vi "SPARK Get Status 0.vi"(8 "error in (no error)":errorcluster, 11 "MotorControlDevRef":T2) -> (0 "error out":errorcluster, 2 "Status 0":T1, 3 "MotorControlDevRef":T2)   [LabVIEW 2023]
uses:
  Typedef/Spark MAX Variant Data.ctl
  Typedef/SPARK Model.ctl
  Typedef/SPARK CAN Arb ID.ctl
  Typedef/SPARK Status 0 Frame.ctl
  <vilib>/Rock Robotics/SystemInterfaces/DIO/FPGA_DIOPWMChannel.ctl
  <vilib>/Rock Robotics/WPI/PWM/WPI_PWMDeadband.ctl
  <vilib>/Rock Robotics/WPI/MotorControl/WPI_MotorControlType.ctl
  <vilib>/Rock Robotics/SystemInterfaces/DIO/FPGA_DIOChannel.ctl
  <vilib>/Rock Robotics/WPI/MotorControl/WPI_MotorControlDeviceRef.ctl
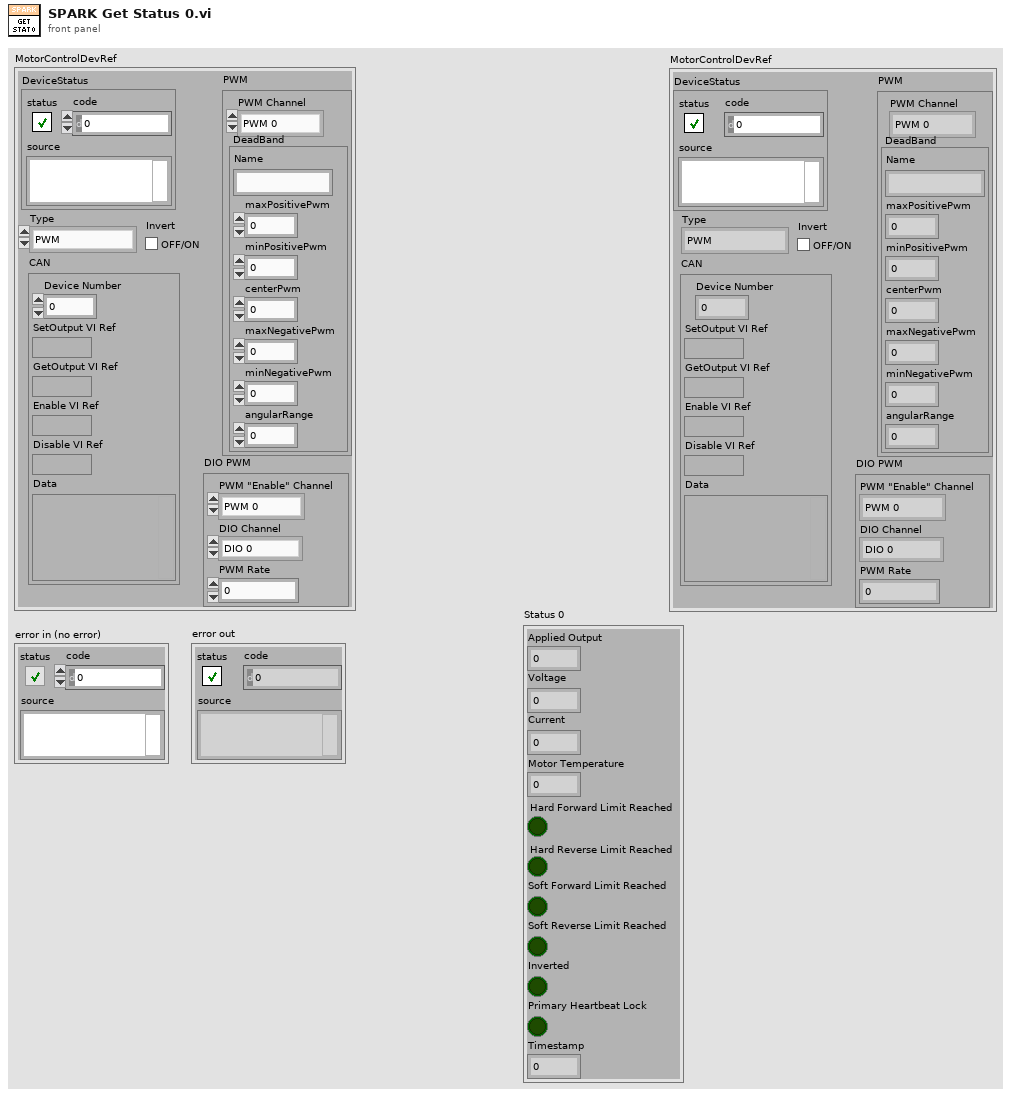
[diagram p1: front panel]
types:
  T1 = typedef "SPARK Status 0 Frame.ctl" = cluster{"Applied Output":dbl, "Voltage":dbl, "Current":dbl, "Motor Temperature":u8, "Hard Forward Limit Reached":bool, "Hard Reverse Limit Reached":bool, "Soft Forward Limit Reached":bool, "Soft Reverse Limit Reached":bool, "Inverted":bool, "Primary Heartbeat Lock":bool, "Timestamp":u32}
  T2 = typedef "WPI_MotorControlDeviceRef.ctl" = cluster{"DeviceStatus":errorcluster, "Type":T3, "PWM":cluster{"PWM Channel":T4, "DeadBand":T5}, "CAN":cluster{"Device Number":u8, "SetOutput VI Ref":variant, "GetOutput VI Ref":variant, "Enable VI Ref":variant, "Disable VI Ref":variant, "Data":variant}, "Invert":bool, "DIO PWM":cluster{"PWM \"Enable\" Channel":T4, "DIOChannel":T6, "PWM Rate":dbl}}
  T3 = typedef "WPI_MotorControlType.ctl" = enum16{"PWM", "CAN", "DIO PWM"}
  T4 = typedef "FPGA_DIOPWMChannel.ctl" = enum8{"PWM 0", "PWM 1", "PWM 2", "PWM 3", "PWM 4", "PWM 5", "PWM 6", "PWM 7", "PWM 8", "PWM 9", "PWM MXP 0", "PWM MXP 1", "PWM MXP 2", "PWM MXP 3", "PWM MXP 4", "PWM MXP 5", "PWM MXP 6", "PWM MXP 7", "PWM MXP 8", "PWM MXP 9", "Invalid"}
  T5 = typedef "WPI_PWMDeadband.ctl" = cluster{"Name":string, "maxPositivePwm":i32, "minPositivePwm":i32, "centerPwm":i32, "maxNegativePwm":i32, "minNegativePwm":i32, "angularRange":u16}
  T6 = typedef "FPGA_DIOChannel.ctl" = enum8{"DIO 0", "DIO 1", "DIO 2", "DIO 3", "DIO 4", "DIO 5", "DIO 6", "DIO 7", "DIO 8", "DIO 9", "DIO MXP 0", "DIO MXP 1", "DIO MXP 2", "DIO MXP 3", "DIO MXP 4", "DIO MXP 5", "DIO MXP 6", "DIO MXP 7", "DIO MXP 8", "DIO MXP 9", "DIO MXP 10", "DIO MXP 11", "DIO MXP 12", "DIO MXP 13", "DIO MXP 14", "DIO MXP 15", "SPI Port CS1", "SPI Port CS2", "SPI Port CS3", "SPI Port MISO", "SPI Port MOSI", "Invalid"}
  T7 = typedef "SPARK CAN Arb ID.ctl" = u32
  T8 = typedef "Spark MAX Variant Data.ctl" = cluster{"Ext ID":u32, "CAN Timeout":u32, "Inverted No WPILib":bool, "Has Configured Limit Sw":bool, "Has Configured Alt Encoder":bool, "SPARK Model":T9, "CAN Max Retries":u32, "CAN Timeout (ms)":u32, "Status 0 Period (ms)":u32, "Status 1 Period (ms)":u32, "Status 2 Period (ms)":u32, "Status 3 Period (ms)":u32, "Status 4 Period (ms)":u32, "Status 5 Period (ms)":u32, "Status 6 Period (ms)":u32, "Status 7 Period (ms)":u32, "Status Frame Timeout (ms)":u32}
  T9 = typedef "SPARK Model.ctl" = enum16{"SPARK MAX", "SPARK Flex", "Unknown"}
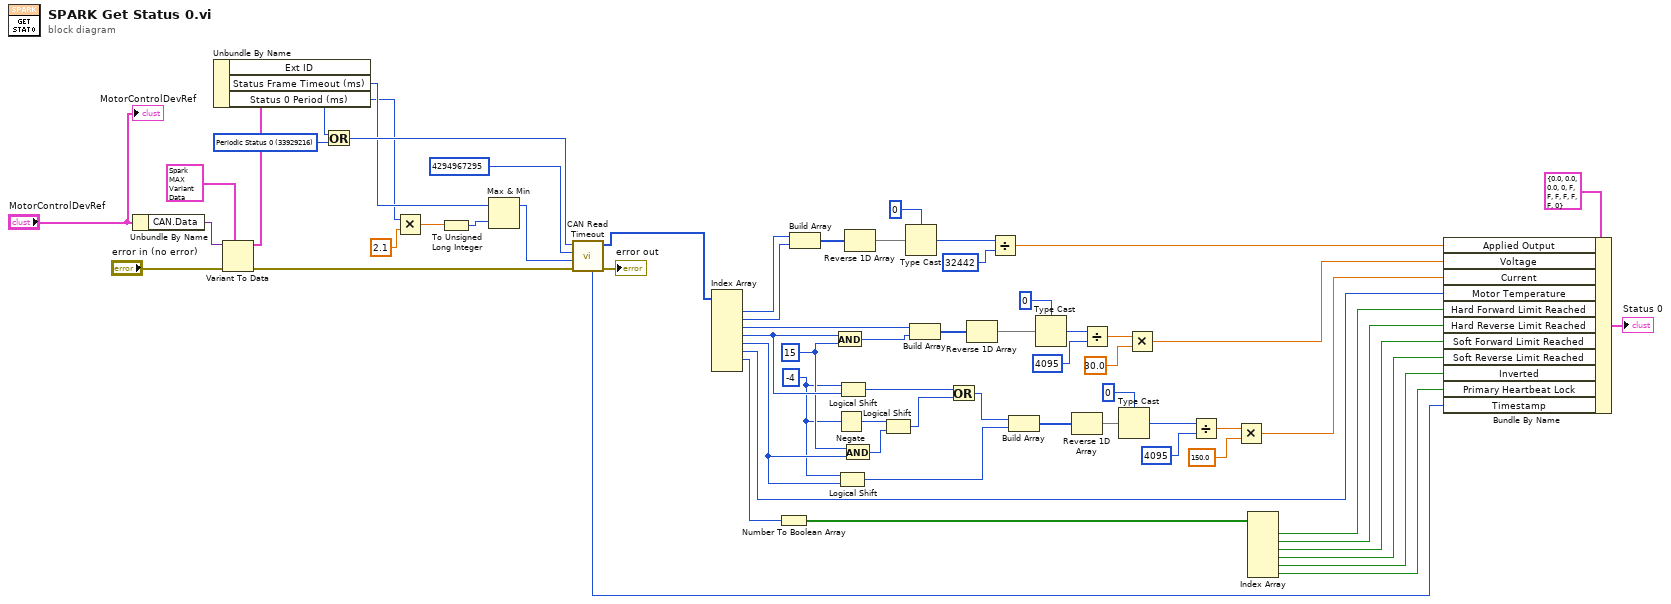
[diagram p0: block diagram]
diagram:
  w1 = i16 -4 ("y")
  w3 = u8 15 ("y")
  w61 = T7 33929216 items=["Broadcast Disable"=0, "Broadcast System Halt"=64, "Broadcast System Reset"=128, "Broadcast Device Assign"=192, "Broadcast Heartbeat"=320, "Broadcast Firmware Version"=512, "Broadcast Enumerate"=576, "Broadcast System Resume"=640, "Velocity Setpoint"=33882112, "Duty Cycle Setpoint"=33882240, "Smart Velocity Setpoint"=33882304, "Position Setpoint"=33882368, "Voltage Setpoint"=33882432, "Current Setpoint"=33882496, "Smart Motion Setpoint"=33882560, "MAXMotion Position Setpoint"=33882624, "MAXMotion Velocity Setpoint"=33882688, "Periodic Status 0"=33929216, "Periodic Status 1"=33929280, "Periodic Status 2"=33929344, "Periodic Status 3"=33929408, "Periodic Status 4"=33929472, "Periodic Status 5"=33929536, "Periodic Status 6"=33929600, "Periodic Status 7"=33929664, "DRV Status"=33888896, "Clear Faults"=33889152, "Parameter Write"=33896448, "Parameter Write Response"=33896512, "Get Config Parameter"=33889344, "Config Burn Flash"=33889408, "Set Follower Mode"=33889472, "Config Factory Defaults"=33889536, "Config Factory Reset"=33889600, "Nack"=33890304, "Ack"=33890368, "Broadcast (not a command)"=33891328, "Heartbeat"=33891456, "Sync"=33891520, "IDQuery"=33891584, "IDAssign"=33891648, "Firmware Version"=33891840, "REV Enumerate"=33891904, "Legacy/USB Heartbeat"=33891968, "roboRIO Lock"=33892032, "SWDL Data"=33892096, "SWDL Checksum"=33892160, "SWDL Retransmit"=33892224, "Telemetry Update Mechanical Position Enoder Port"=33892352, "Telemetry Update I Accum"=33892480, "Telemtry Update Mechanical Position Alt Encoder"=33892608, "Telemetry Update Mechanical Position Analog"=33892544, "Non-roboRIO Broadcast (not a command)"=33893376, "non-RIO Lock"=33893440, "non-RIO Heartbeat"=33893504] ("SPARK Arb ID")
  n1 = Unbundle By Name("MotorControlDevRef") -> ("CAN.Data"=w64:variant)
  n2 = Variant To Data(error in="error in (no error)", type=T8 {"Ext ID"=0, "CAN Timeout"=0, "Inverted No WPILib"=FALSE, "Has Configured Limit Sw"=FALSE, "Has Configured Alt Encoder"=FALSE, "SPARK Model"=enum."Unknown", "CAN Max Retries"=5, "CAN Timeout (ms)"=20, "Status 0 Period (ms)"=10, "Status 1 Period (ms)"=250, "Status 2 Period (ms)"=20, "Status 3 Period (ms)"=20, "Status 4 Period (ms)"=20, "Status 5 Period (ms)"=20, "Status 6 Period (ms)"=20, "Status 7 Period (ms)"=20, "Status Frame Timeout (ms)"=500} ("SPARK TNG Device Ref"), Variant=w64) -> (data=w56:T8, error out=w58:errorcluster)
  n3 = Unbundle By Name(w56) -> ("Ext ID"=w62:u32, "Status Frame Timeout (ms)"=w20:u32, "Status 0 Period (ms)"=w19:u32)
  n4 = Or(x=w62, y=w61) -> (x .or. y?=w60:T7)
  n5 = Multiply(x=w19, y=2.1) -> (x*y=w17:dbl)
  n6 = To Unsigned Long Integer(number=w17) -> (unsigned 32bit integer=w16:u32)
  n7 = Max & Min(x=w20, y=w16) -> (max(x,y)=w15:u32)  [unwired: 1 out]
  n8 = call "CAN Read Timeout.vi"("error in (no error)"=w58, "Timeout (ms)"=w15, "Message ID Mask"=u32 4294967295, "Message ID"=w60) -> ("error out"=→"error out":errorcluster, "data"=w48:u8[], "timestamp"=w29:u32)  [unwired: 5 in]
  n9 = Index Array(array=w48) -> (element #1=w47:u8, element #2=w46:u8, element #3=w44:u8, element #4=w14:u8, element #5=w5:u8, element #6=w10:u8, element #7=w13:u8)  [unwired: 8 in, 1 out]
  n10 = Number To Boolean Array(number=w13) -> (Boolean array=w28:bool[])
  n11 = Build Array(w47, w46) -> (w45:u8[])
  n12 = And(x=w14, y=w3) -> (x .and. y?=w42:u8)
  n13 = Negate(x=w1) -> (-x=w2:i16)
  n14 = Logical Shift(y=w1, x=w5) -> (x << y=w4:u8)
  n15 = Logical Shift(y=w1, x=w14) -> (x << y=w9:u8)
  n16 = And(x=w3, y=w5) -> (x .and. y?=w7:u8)
  n17 = Reverse 1D Array(array=w45) -> (reversed array=w53:u8[])
  n18 = Logical Shift(y=w2, x=w7) -> (x << y=w6:u8)
  n19 = Type Cast(type=i16 0, x=w53) -> (*(type *) &x=w51:i16)
  n20 = Build Array(w44, w42) -> (w43:u8[])
  n21 = Or(x=w9, y=w6) -> (x .or. y?=w8:u8)
  n22 = Reverse 1D Array(array=w43) -> (reversed array=w40:u8[])
  n23 = Divide(x=w51, y=i16 32442) -> (x/y=w49:dbl)
  n24 = Build Array(w8, w4) -> (w12:u8[])
  n25 = Type Cast(type=i16 0, x=w40) -> (*(type *) &x=w39:i16)
  n26 = Reverse 1D Array(array=w12) -> (reversed array=w11:u8[])
  n27 = Divide(x=w39, y=i16 4095) -> (x/y=w37:dbl)
  n28 = Type Cast(type=i16 0, x=w11) -> (*(type *) &x=w31:i16)
  n29 = Multiply(x=w37, y=30.0) -> (x*y=w21:dbl)
  n30 = Divide(x=w31, y=i16 4095) -> (x/y=w33:dbl)
  n31 = Multiply(x=w33, y=150.0) -> (x*y=w30:dbl)
  n32 = Index Array(array=w28) -> (element #1=w27:bool, element #2=w26:bool, element #3=w25:bool, element #4=w24:bool, element #5=w23:bool, element #6=w22:bool)  [unwired: 6 in]
  n33 = Bundle By Name(cluster=T1 {"Applied Output"=0.0, "Voltage"=0.0, "Current"=0.0, "Motor Temperature"=0, "Hard Forward Limit Reached"=FALSE, "Hard Reverse Limit Reached"=FALSE, "Soft Forward Limit Reached"=FALSE, "Soft Reverse Limit Reached"=FALSE, "Inverted"=FALSE, "Primary Heartbeat Lock"=FALSE, "Timestamp"=0} ("SPARK Status 0"), "Applied Output"=w49, "Voltage"=w21, "Current"=w30, "Motor Temperature"=w10, "Hard Forward Limit Reached"=w27, "Hard Reverse Limit Reached"=w26, "Soft Forward Limit Reached"=w25, "Soft Reverse Limit Reached"=w24, "Inverted"=w23, "Primary Heartbeat Lock"=w22, "Timestamp"=w29) -> (→"Status 0":T1)
  "MotorControlDevRef" <- "MotorControlDevRef"
